vi "Amplitude_Shift_Keying.vi"() -> ()   [LabVIEW 2019]
panel:
  out "Modulated Signal":dbl[](graph)=[0.0, 0.5877852522924731, 0.9510565162951535, 0.9510565162951536, 0.5877852522924732, 1.2246467991473532e-16, -0.5877852522924727, -0.9510565162951535, -0.9510565162951536, -0.587785252292474, -2.4492935982947064e-16, 0.5877852522924729, 0.9510565162951532, 0.9510565162951542, 0.5877852522924734, 3.6739403974420594e-16, -0.5877852522924728, -0.9510565162951529, -0.9510565162951543, -0.5877852522924735, -4.898587196589413e-16, 0.5877852522924712, 0.9510565162951534, 0.9510565162951543, 0.587785252292475, 6.123233995736766e-16, -0.5877852522924697, -0.9510565162951534, -0.9510565162951538, -0.5877852522924766, -7.347880794884119e-16, 0.5877852522924696, 0.9510565162951533, 0.9510565162951539, 0.5877852522924767, 8.572527594031472e-16, -0.5877852522924696, -0.9510565162951533, -0.9510565162951539, -0.5877852522924768, -9.797174393178826e-16, 0.5877852522924724, 0.9510565162951522, 0.9510565162951539, 0.587785252292474, 4.654895798033119e-15, -0.5877852522924694, -0.9510565162951532, -0.9510565162951551, -0.587785252292477, -1.2246467991473533e-15, 0.587785252292475, 0.951056516295151, 0.9510565162951551, 0.5877852522924742, 4.899825157862589e-15, -0.587785252292472, -0.9510565162951521, -0.9510565162951562, -0.5877852522924771, -1.4695761589768238e-15, 0.5877852522924748, 0.9510565162951509, 0.9510565162951552, 0.5877852522924744, 5.14475451769206e-15, -0.5877852522924718, -0.951056516295152, -0.9510565162951563, -0.5877852522924774, -1.7145055188062944e-15, 0.5877852522924688, 0.9510565162951509, 0.9510565162951552, 0.5877852522924746, 5.3896838775215305e-15, -0.5877852522924716, -0.9510565162951519, -0.9510565162951563, -0.5877852522924718, -1.959434878635765e-15, 0.5877852522924687, 0.951056516295153, 0.9510565162951553, 0.5877852522924806, -1.4708141202500005e-15, -0.5877852522924714, -0.9510565162951496, -0.9510565162951542, -0.5877852522924778, -9.309791596066238e-15, 0.5877852522924685, 0.9510565162951506, 0.9510565162951575, 0.587785252292475, 5.879542597180472e-15, -0.5877852522924655, -0.9510565162951518, -0.9510565162951565, -0.5877852522924722, -2.4492935982947065e-15, 0.5877852522924683, 0.951056516295155, 0.9510565162951554, 0.5877852522924867, -9.809554005910593e-16, -0.5877852522924653, -0.9510565162951516, -0.9510565162951544, -0.5877852522924839, -9.799650315725178e-15, 0.587785252292468, 0.9510565162951528, 0.9510565162951578, 0.5877852522924811, 6.369401316839413e-15, -0.5877852522924594, -0.9510565162951538, -0.9510565162951566, -0.5877852522924784, -2.9391523179536475e-15, 0.5877852522924621, 0.9510565162951549, 0.9510565162951556, 0.5877852522924871, -4.91096680932118e-16, -0.5877852522924649, -0.9510565162951515, -0.9510565162951545, -0.5877852522924844, -1.028950903538412e-14, 0.5877852522924677, 0.9510565162951525, 0.9510565162951579, 0.5877852522924816, 6.859260036498355e-15, -0.5877852522924589, -0.9510565162951536, -0.9510565162951569, -0.5877852522924902, -3.429011037612589e-15, 0.5877852522924617, 0.9510565162951503, 0.9510565162951558, 0.5877852522924875, -1.2379612731767154e-18, -0.5877852522924645, -0.9510565162951513, -0.9510565162951546, -0.5877852522924847, -1.0779367755043061e-14, 0.5877852522924673, 0.9510565162951524, 0.951056516295158, 0.5877852522924819, 7.349118756157295e-15, -0.5877852522924585, -0.9510565162951491, -0.9510565162951525, -0.5877852522924791, -3.91886975727153e-15, 0.5877852522924614, 0.9510565162951502, 0.9510565162951603, 0.5877852522924764, 4.886207583857646e-16, -0.587785252292464, -0.9510565162951512, -0.9510565162951592, -0.5877852522924851, 2.941628240500001e-15, 0.5877852522924669, 0.9510565162951523, 0.9510565162951582, 0.5877852522924938, 7.838977475816237e-15, -0.5877852522924696, -0.951056516295149, -0.9510565162951571, -0.587785252292491, -1.8619583192132475e-14, 0.5877852522924725, 0.95105651629515, 0.9510565162951561, 0.5877852522924882, 1.518933419324671e-14, -0.5877852522924522, -0.9510565162951511, -0.951056516295155, -0.5877852522924855, -1.1759085194360944e-14, 0.5877852522924549, 0.9510565162951478, 0.951056516295154, 0.5877852522924827, 8.328836195475178e-15, -0.5877852522924577, -0.9510565162951488, -0.9510565162951529, -0.5877852522924799, -4.898587196589413e-15, 0.5877852522924605, 0.9510565162951499, 0.9510565162951606, 0.5877852522924657, 1.567919291290565e-14, -0.5877852522924633, -0.9510565162951509, -0.951056516295164, -0.5877852522924973, 1.9619108011821185e-15, 0.5877852522924546, 0.9510565162951475, 0.9510565162951585, 0.5877852522924831, 3.7240404345538126e-14, -0.5877852522924688, -0.951056516295153, -0.9510565162951619, -0.5877852522924918, -1.9599300631450357e-14, 0.5877852522924601, 0.9510565162951496, 0.9510565162951563, 0.5877852522924776, 3.0379906347766594e-14, -0.5877852522924514, -0.9510565162951552, -0.0, -0.0, -0.0, 0.0, 0.0, 0.0, 0.0, 0.0, -0.0, -0.0, -0.0, -0.0, -0.0, 0.0, 0.0, 0.0, 0.0, 0.0, -0.0, -0.0, -0.0, -0.0, 0.0, 0.0, 0.0, 0.0, 0.0, 0.0, -0.0, -0.0, -0.0, -0.0, -0.0, 0.0, 0.0, 0.0, 0.0, 0.0, -0.0, -0.0, -0.0, -0.0, -0.0, 0.0, 0.0, 0.0, 0.0, 0.0, -0.0, -0.0, -0.0, -0.0, -0.0, 0.0, 0.0, 0.0, 0.0, 0.0, -0.0, -0.0, -0.0, -0.0, 0.0, 0.0, 0.0, 0.0, 0.0, 0.0, -0.0, -0.0, -0.0, -0.0, -0.0, 0.0, 0.0, 0.0, 0.0, 0.0, -0.0, -0.0, -0.0, -0.0, -0.0, 0.0, 0.0, 0.0, 0.0, 0.0, -0.0, -0.0, -0.0, -0.0, -0.0, 0.0, 0.0, 0.0, 0.0, 0.0, -0.0, -0.0, -0.0, -0.0, -0.0, 0.0, 0.0, 0.0, 0.0, 0.0, -0.0, -0.0, -0.0, -0.0, 0.0, 0.0, 0.0, 0.0, 0.0, 0.0, -0.0, -0.0, -0.0, -0.0, -0.0, 0.0, 0.0, 0.0, 0.0, 0.0, -0.0, -0.0, -0.0, -0.0, -0.0, 0.0, 0.0, 0.0, 0.0, 0.0, -0.0, -0.0, -0.0, -0.0, -0.0, 0.0, 0.0, 0.0, 0.0, 0.0, -0.0, -0.0, -0.0, -0.0, -0.0, 0.0, 0.0, 0.0, 0.0, 0.0, -0.0, -0.0, -0.0, -0.0, -0.0, 0.0, 0.0, 0.0, 0.0, 0.0, -0.0, -0.0, -0.0, -0.0, -0.0, 0.0, 0.0, 0.0, 0.0, 0.0, -0.0, -0.0, -0.0, -0.0, -0.0, 0.0, 0.0, 0.0, 0.0, -0.0, -0.0, -0.0, -0.0, -0.0, 0.0, 0.0, 0.0, 0.0, 0.0, 0.0, -0.0, -0.0, -0.0, -0.0, -0.0, 0.0, 0.0, 0.0, 0.0, 0.0, -0.0, -0.0, -0.0, -0.0, -0.0, 0.0, 0.0, 0.0, 0.0, 0.0, -0.0, -0.0, -0.0, -0.0, -0.0, 0.0, 0.0, 0.0, 0.0]
  out "Carrier Signal":dbl[](graph)=[0.0, 0.5877852522924731, 0.9510565162951535, 0.9510565162951536, 0.5877852522924732, 1.2246467991473532e-16, -0.5877852522924727, -0.9510565162951535, -0.9510565162951536, -0.587785252292474, -2.4492935982947064e-16, 0.5877852522924729, 0.9510565162951532, 0.9510565162951542, 0.5877852522924734, 3.6739403974420594e-16, -0.5877852522924728, -0.9510565162951529, -0.9510565162951543, -0.5877852522924735, -4.898587196589413e-16, 0.5877852522924712, 0.9510565162951534, 0.9510565162951543, 0.587785252292475, 6.123233995736766e-16, -0.5877852522924697, -0.9510565162951534, -0.9510565162951538, -0.5877852522924766, -7.347880794884119e-16, 0.5877852522924696, 0.9510565162951533, 0.9510565162951539, 0.5877852522924767, 8.572527594031472e-16, -0.5877852522924696, -0.9510565162951533, -0.9510565162951539, -0.5877852522924768, -9.797174393178826e-16, 0.5877852522924724, 0.9510565162951522, 0.9510565162951539, 0.587785252292474, 4.654895798033119e-15, -0.5877852522924694, -0.9510565162951532, -0.9510565162951551, -0.587785252292477, -1.2246467991473533e-15, 0.587785252292475, 0.951056516295151, 0.9510565162951551, 0.5877852522924742, 4.899825157862589e-15, -0.587785252292472, -0.9510565162951521, -0.9510565162951562, -0.5877852522924771, -1.4695761589768238e-15, 0.5877852522924748, 0.9510565162951509, 0.9510565162951552, 0.5877852522924744, 5.14475451769206e-15, -0.5877852522924718, -0.951056516295152, -0.9510565162951563, -0.5877852522924774, -1.7145055188062944e-15, 0.5877852522924688, 0.9510565162951509, 0.9510565162951552, 0.5877852522924746, 5.3896838775215305e-15, -0.5877852522924716, -0.9510565162951519, -0.9510565162951563, -0.5877852522924718, -1.959434878635765e-15, 0.5877852522924687, 0.951056516295153, 0.9510565162951553, 0.5877852522924806, -1.4708141202500005e-15, -0.5877852522924714, -0.9510565162951496, -0.9510565162951542, -0.5877852522924778, -9.309791596066238e-15, 0.5877852522924685, 0.9510565162951506, 0.9510565162951575, 0.587785252292475, 5.879542597180472e-15, -0.5877852522924655, -0.9510565162951518, -0.9510565162951565, -0.5877852522924722, -2.4492935982947065e-15, 0.5877852522924683, 0.951056516295155, 0.9510565162951554, 0.5877852522924867, -9.809554005910593e-16, -0.5877852522924653, -0.9510565162951516, -0.9510565162951544, -0.5877852522924839, -9.799650315725178e-15, 0.587785252292468, 0.9510565162951528, 0.9510565162951578, 0.5877852522924811, 6.369401316839413e-15, -0.5877852522924594, -0.9510565162951538, -0.9510565162951566, -0.5877852522924784, -2.9391523179536475e-15, 0.5877852522924621, 0.9510565162951549, 0.9510565162951556, 0.5877852522924871, -4.91096680932118e-16, -0.5877852522924649, -0.9510565162951515, -0.9510565162951545, -0.5877852522924844, -1.028950903538412e-14, 0.5877852522924677, 0.9510565162951525, 0.9510565162951579, 0.5877852522924816, 6.859260036498355e-15, -0.5877852522924589, -0.9510565162951536, -0.9510565162951569, -0.5877852522924902, -3.429011037612589e-15, 0.5877852522924617, 0.9510565162951503, 0.9510565162951558, 0.5877852522924875, -1.2379612731767154e-18, -0.5877852522924645, -0.9510565162951513, -0.9510565162951546, -0.5877852522924847, -1.0779367755043061e-14, 0.5877852522924673, 0.9510565162951524, 0.951056516295158, 0.5877852522924819, 7.349118756157295e-15, -0.5877852522924585, -0.9510565162951491, -0.9510565162951525, -0.5877852522924791, -3.91886975727153e-15, 0.5877852522924614, 0.9510565162951502, 0.9510565162951603, 0.5877852522924764, 4.886207583857646e-16, -0.587785252292464, -0.9510565162951512, -0.9510565162951592, -0.5877852522924851, 2.941628240500001e-15, 0.5877852522924669, 0.9510565162951523, 0.9510565162951582, 0.5877852522924938, 7.838977475816237e-15, -0.5877852522924696, -0.951056516295149, -0.9510565162951571, -0.587785252292491, -1.8619583192132475e-14, 0.5877852522924725, 0.95105651629515, 0.9510565162951561, 0.5877852522924882, 1.518933419324671e-14, -0.5877852522924522, -0.9510565162951511, -0.951056516295155, -0.5877852522924855, -1.1759085194360944e-14, 0.5877852522924549, 0.9510565162951478, 0.951056516295154, 0.5877852522924827, 8.328836195475178e-15, -0.5877852522924577, -0.9510565162951488, -0.9510565162951529, -0.5877852522924799, -4.898587196589413e-15, 0.5877852522924605, 0.9510565162951499, 0.9510565162951606, 0.5877852522924657, 1.567919291290565e-14, -0.5877852522924633, -0.9510565162951509, -0.951056516295164, -0.5877852522924973, 1.9619108011821185e-15, 0.5877852522924546, 0.9510565162951475, 0.9510565162951585, 0.5877852522924831, 3.7240404345538126e-14, -0.5877852522924688, -0.951056516295153, -0.9510565162951619, -0.5877852522924918, -1.9599300631450357e-14, 0.5877852522924601, 0.9510565162951496, 0.9510565162951563, 0.5877852522924776, 3.0379906347766594e-14, -0.5877852522924514, -0.9510565162951552, -0.9510565162951596, -0.5877852522924862, -1.2738802633678827e-14, 0.5877852522924657, 0.951056516295143, 0.9510565162951542, 0.587785252292472, 2.3519408349995066e-14, -0.5877852522924569, -0.9510565162951485, -0.9510565162951575, -0.5877852522924807, -5.878304635907295e-15, 0.5877852522924712, 0.9510565162951452, 0.9510565162951609, 0.5877852522924665, 1.6658910352223535e-14, -0.5877852522924625, -0.9510565162951506, -0.9510565162951642, -0.5877852522924982, 9.82193361864236e-16, 0.5877852522924538, 0.9510565162951473, 0.9510565162951587, 0.5877852522924839, 3.822012178485601e-14, -0.587785252292468, -0.9510565162951528, -0.9510565162951621, -0.5877852522924927, -2.057901807076824e-14, 0.5877852522924594, 0.9510565162951494, 0.9510565162951566, 0.5877852522924784, 3.1359623787084476e-14, -0.5877852522924506, -0.9510565162951549, -0.95105651629516, -0.5877852522924871, -1.371852007299671e-14, 0.5877852522924649, 0.9510565162951428, 0.9510565162951545, 0.5877852522924728, 2.4499125789312947e-14, -0.5877852522924562, -0.9510565162951482, -0.9510565162951666, -0.5877852522924816, -6.858022075225178e-15, 0.5877852522924474, 0.9510565162951449, 0.9510565162951612, 0.5877852522924902, 1.7638627791541416e-14, -0.5877852522924617, -0.9510565162951503, -0.9510565162951645, -0.587785252292499, 2.475922546353431e-18, 0.5877852522924529, 0.951056516295147, 0.9510565162951591, 0.5877852522924847, 3.9199839224173895e-14, -0.5877852522924673, -0.9510565162951524, -0.9510565162951624, -0.5877852522924935, -2.1558735510086122e-14, 0.5877852522924585, 0.9510565162951491, 0.951056516295157, 0.5877852522924791, 3.2339341226402363e-14, -0.5877852522924498, -0.9510565162951545, -0.9510565162951603, -0.5877852522924879, -1.469823751231459e-14, 0.587785252292464, 0.9510565162951424, 0.9510565162951549, 0.5877852522924966, 2.547884322863083e-14, -0.5877852522924784, -0.9510565162951479, -0.9510565162951582, -0.5877852522925053, -7.83773951454306e-15, 0.5877852522924466, 0.9510565162951445, 0.9510565162951528, 0.587785252292491, 1.8618345230859297e-14, -0.5877852522924379, -0.95105651629515, -0.9510565162951561, -0.5877852522924998, -9.772415167715292e-16, 0.5877852522924522, 0.9510565162951466, 0.9510565162951506, 0.5877852522924855, 1.1757847233087767e-14, -0.5877852522924435, -0.9510565162951521, -0.9510565162951627, -0.5877852522924942, 5.883256481000002e-15, 0.5877852522924577, 0.9510565162951488, 0.9510565162951661, 0.5877852522924799, 4.897349235316236e-15, -0.587785252292449, -0.9510565162951542, -0.9510565162951694, -0.5877852522924887, -1.5677954951632475e-14, 0.5877852522924403, 0.9510565162951509, 0.951056516295164, 0.5877852522924973, 5.488027009835272e-14, -0.5877852522924546, -0.9510565162951475, -0.9510565162951673, -0.5877852522924831, -3.723916638426495e-14, 0.5877852522924458, 0.951056516295153, 0.9510565162951619, 0.5877852522924918, 4.801977210058119e-14, -0.5877852522924601, -0.9510565162951496, -0.9510565162951652, -0.5877852522924776, -3.037866838649342e-14, 0.5877852522924514, 0.9510565162951375, 0.9510565162951596, 0.5877852522924862, 4.115927410280966e-14, -0.5877852522924657, -0.951056516295143, -0.951056516295163, -0.587785252292472, -2.3518170388721888e-14, 0.5877852522924569, 0.9510565162951397, 0.9510565162951575, 0.5877852522925038, 3.4298776105038126e-14, -0.5877852522924712, -0.9510565162951452, -0.9510565162951609, -0.5877852522925124, -1.6657672390950356e-14, 0.5877852522924625, 0.9510565162951419, 0.9510565162951554, 0.5877852522924982, 2.7438278107266594e-14, -0.5877852522924768, -0.9510565162951473, -0.9510565162951587, -0.5877852522925069, -9.797174393178826e-15, 0.587785252292445, 0.951056516295144, 0.9510565162951533, 0.5877852522924927, 2.0577780109495062e-14, -0.5877852522924364, -0.9510565162951494, -0.9510565162951479, -0.5877852522924784, -3.13583858258113e-14, 0.5877852522924276, 0.9510565162951461, 0.9510565162951512, 0.5877852522924871, -1.4704427318680477e-14, -0.587785252292419, -0.9510565162951428, -0.9510565162951721, -0.5877852522924958, 3.923821602364237e-15, 0.5877852522924562, 0.9510565162951394, 0.9510565162951754, 0.5877852522925046, 6.856784113952001e-15, -0.5877852522924474, -0.9510565162951536, -0.9510565162951612, -0.5877852522925132, -7.448080869107625e-14, 0.5877852522924387, 0.9510565162951503, 0.9510565162951645, 0.587785252292476, 2.8417995546584478e-14, -0.58778525229243, -0.951056516295147, -0.9510565162951679, -0.5877852522924847, -3.919860126290071e-14, 0.5877852522924673, 0.9510565162951437, 0.9510565162951712, 0.5877852522924935, 4.997920697921695e-14, -0.5877852522924585, -0.9510565162951403, -0.951056516295157, -0.5877852522925021, -6.075981269553319e-14, 0.5877852522924498, 0.951056516295137, 0.9510565162951603, 0.5877852522924649]
  out "Modulating Signal":i16[](graph)=[0, 1, 1, 1, 1, 1, 1, 1, 1, 1, 1, 1, 1, 1, 1, 1, 1, 1, 1, 1, 1, 1, 1, 1, 1, 1, 1, 1, 1, 1, 1, 1, 1, 1, 1, 1, 1, 1, 1, 1, 1, 1, 1, 1, 1, 1, 1, 1, 1, 1, 1, 1, 1, 1, 1, 1, 1, 1, 1, 1, 1, 1, 1, 1, 1, 1, 1, 1, 1, 1, 1, 1, 1, 1, 1, 1, 1, 1, 1, 1, 1, 1, 1, 1, 1, 1, 1, 1, 1, 1, 1, 1, 1, 1, 1, 1, 1, 1, 1, 1, 1, 1, 1, 1, 1, 1, 1, 1, 1, 1, 1, 1, 1, 1, 1, 1, 1, 1, 1, 1, 1, 1, 1, 1, 1, 1, 1, 1, 1, 1, 1, 1, 1, 1, 1, 1, 1, 1, 1, 1, 1, 1, 1, 1, 1, 1, 1, 1, 1, 1, 1, 1, 1, 1, 1, 1, 1, 1, 1, 1, 1, 1, 1, 1, 1, 1, 1, 1, 1, 1, 1, 1, 1, 1, 1, 1, 1, 1, 1, 1, 1, 1, 1, 1, 1, 1, 1, 1, 1, 1, 1, 1, 1, 1, 1, 1, 1, 1, 1, 1, 1, 1, 1, 1, 1, 1, 1, 1, 1, 1, 1, 1, 1, 1, 1, 1, 1, 1, 1, 1, 1, 1, 1, 1, 1, 1, 1, 1, 0, 0, 0, 0, 0, 0, 0, 0, 0, 0, 0, 0, 0, 0, 0, 0, 0, 0, 0, 0, 0, 0, 0, 0, 0, 0, 0, 0, 0, 0, 0, 0, 0, 0, 0, 0, 0, 0, 0, 0, 0, 0, 0, 0, 0, 0, 0, 0, 0, 0, 0, 0, 0, 0, 0, 0, 0, 0, 0, 0, 0, 0, 0, 0, 0, 0, 0, 0, 0, 0, 0, 0, 0, 0, 0, 0, 0, 0, 0, 0, 0, 0, 0, 0, 0, 0, 0, 0, 0, 0, 0, 0, 0, 0, 0, 0, 0, 0, 0, 0, 0, 0, 0, 0, 0, 0, 0, 0, 0, 0, 0, 0, 0, 0, 0, 0, 0, 0, 0, 0, 0, 0, 0, 0, 0, 0, 0, 0, 0, 0, 0, 0, 0, 0, 0, 0, 0, 0, 0, 0, 0, 0, 0, 0, 0, 0, 0, 0, 0, 0, 0, 0, 0, 0, 0, 0, 0, 0, 0, 0, 0, 0, 0, 0, 0, 0, 0, 0, 0, 0, 0, 0, 0, 0, 0, 0, 0, 0, 0, 0, 0, 0, 0, 0, 0, 0, 0, 0, 0, 0, 0, 0, 0, 0, 0, 0, 0, 0, 0, 0, 0, 0, 0, 0, 0, 0, 0, 0, 0, 0, 0, 0, 0, 0, 0, 0, 0, 0, 0, 0, 0, 0, 0, 0, 0, 0, 0]
  in  "fm":dbl=11.0
  out "No. of\nsamples":dbl=454.54545454545456
  in  "No. of\ncycles":dbl=1.0
  in  "fs":dbl=5000.0
  in  "fc":dbl=500.0
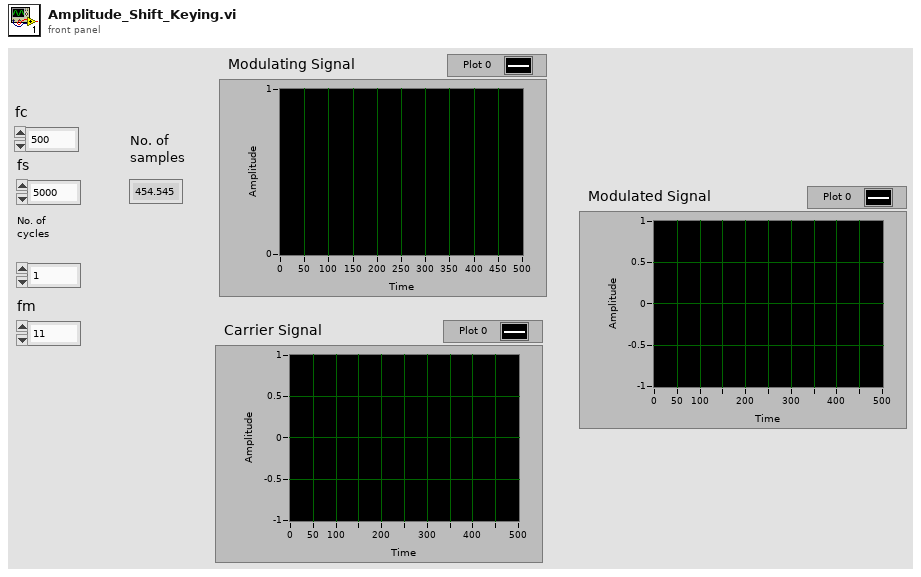
[diagram p1: front panel]
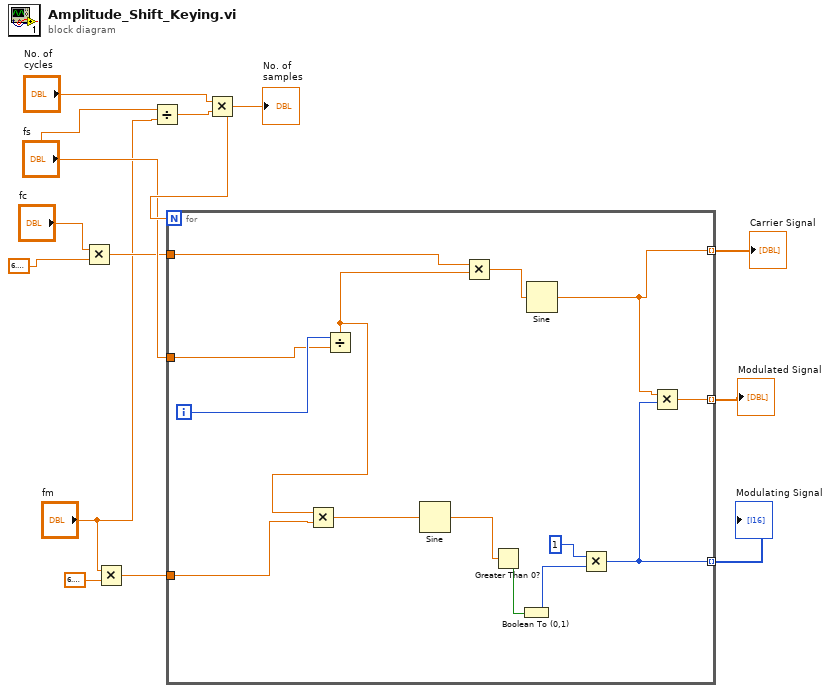
[diagram p0: block diagram]
diagram:
  n1 = Multiply(x="fc", y=6.283185307179586) -> (x*y=w6:dbl)
  n2 = Multiply(x="fm", y=6.283185307179586) -> (x*y=w7:dbl)
  n3 = Divide(x="fs", y="fm") -> (x/y=w13:dbl)
  n4 = Multiply(x="No. of\ncycles", y=w13) -> (x*y=w11:dbl)
  "No. of\nsamples" <- w11
  n5 = for {
    N: w11 -> [_]
    tunnel: "fs" -> [w26]
    tunnel: w7 -> [w25]
    tunnel: w6 -> [w22]
    tunnel: [w16] -> w3 mode=indexing
    tunnel: [w14] -> w2 mode=indexing
    tunnel: [w15] -> w1 mode=indexing
    i -> [w27]
    n6 = Divide(x=w27, y=w26) -> (x/y=w21:dbl)
    n7 = Multiply(x=w21, y=w25) -> (x*y=w24:dbl)
    n8 = Sine(x=w24) -> (sin(x)=w20:dbl)
    n9 = Multiply(x=w22, y=w21) -> (x*y=w23:dbl)
    n10 = Greater Than 0?(x=w20) -> (x > 0?=w19:bool)
    n11 = Boolean To (0,1)(Boolean=w19) -> (0, 1=w18:i16)
    n12 = Sine(x=w23) -> (sin(x)=w16:dbl)
    n13 = Multiply(x=i16 1, y=w18) -> (x*y=w14:i16)
    n14 = Multiply(x=w16, y=w14) -> (x*y=w15:dbl)
  }
  "Modulating Signal" <- w2
  "Carrier Signal" <- w3
  "Modulated Signal" <- w1
